vi "Logarithm of Factorial.vi"(3 "n":i32) -> (1 "ln(n!)":dbl format="%.2f")   [LabVIEW 2020, in "NI_Gmath.lvlib"]
doc: "Computes the natural logarithm of a factorial."
uses:
  <vilib>/gmath/NI_Gmath.lvlib
  <resource>/lvanlys.dll
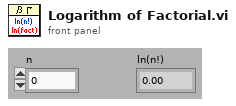
[diagram p1: front panel]
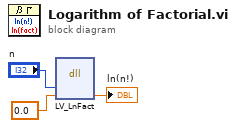
[diagram p0: block diagram]
diagram:
  n1 = dll-call lib="e:/builds/penguin/labview/branches/2020/dev/dist/resource/lvanlys.*" fn="LV_LnFact"("n"="n", "ln(n!)"=0.0 ("factorial")) -> ("ln(n!)"=→"ln(n!)":dbl)  [unwired: 5 in, 2 out]
